vi "click.vi"(8 "error in (no error)":errorcluster, 10 "Control Label":string, 11 "VI Ref":refnum<vi>) -> (0 "error out":errorcluster, 3 "return value":string)   [LabVIEW 2020]
uses:
  ui-testing.lvlib
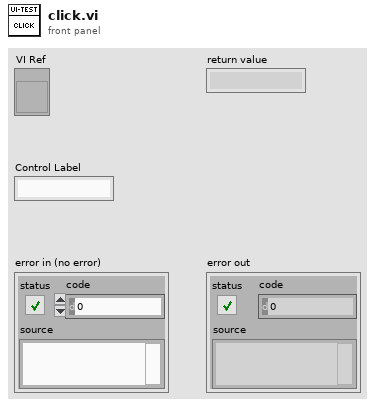
[diagram p1: front panel]
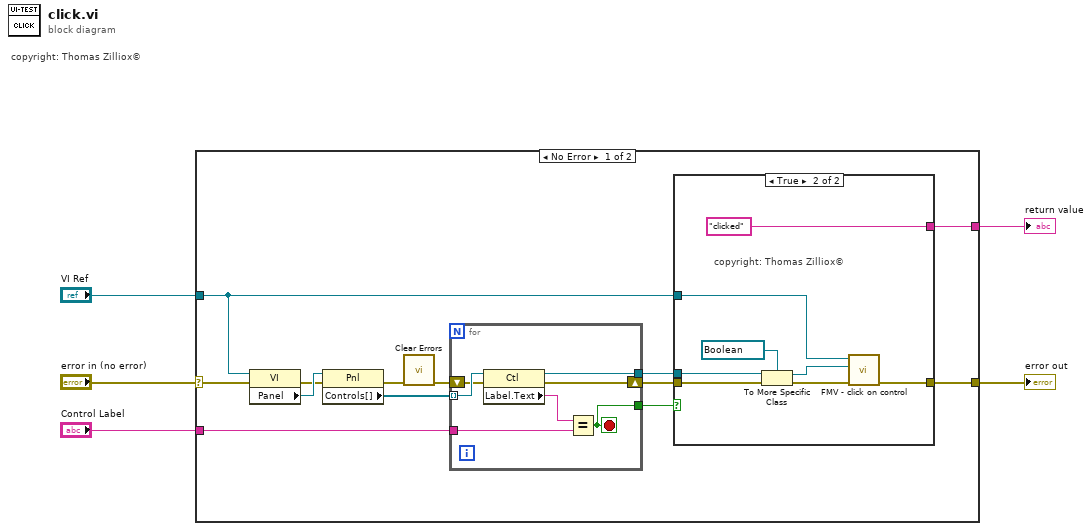
[diagram p0: block diagram]
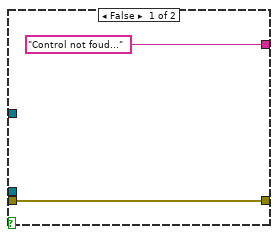
[diagram p2: hidden frame]
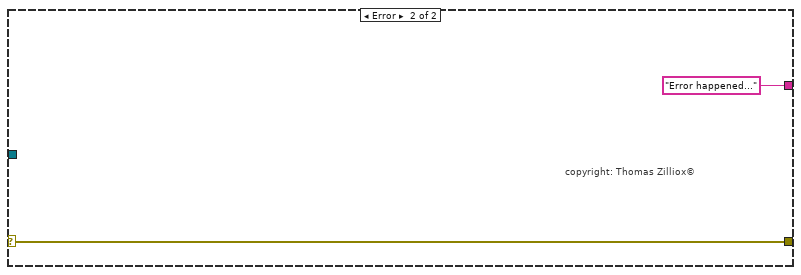
[diagram p3: hidden frame]
diagram:
  # "copyright: Thomas Zilliox©"
  n1 = case shown="No Error" "error in (no error)" {
    selector: "error in (no error)" -> [w13 w37]
    tunnel: [w11 w37] -> w4
    tunnel: "Control Label" -> [w12 _]
    tunnel: [w7 "Error happened..."] -> w2
    tunnel: "VI Ref" -> [w6 _]
    frame No Error {
      n2 = property class="VI"(reference=w6, error in=w13) -> (error out=w16:errorcluster, "Panel"=w18:refnum<vi>)  [unwired: 1 out]
      n3 = property class="Pnl"(reference=w18, error in=w16) -> (error out=w15:errorcluster, "Controls[]"=w17:refnum<vi>[])  [unwired: 1 out]
      n4 = call <vilib>:"Clear Errors.vi"("error in (no error)"=w15) -> ("error out"=w10:errorcluster)  [unwired: 5 in, 1 out]
      n5 = for {
        tunnel: w17 -> [w35] mode=indexing
        tunnel: w12 -> [w33]
        tunnel: [w32] -> w14
        shift-right: [w30] -> w9
        shift-left: w10 -> [w31]
        tunnel: [w29] -> w8
        stop <- w29 stop-if-true
        n6 = property class="Ctl"(reference=w35, error in=w31) -> (reference out=w32:refnum<vi>, error out=w30:errorcluster, "Label.Text"=w34:string)
        n7 = Equal?(x=w34, y=w33) -> (x = y?=w29:bool)
      }
      n8 = case shown="True" w8 {
        tunnel: w14 -> [_ w28]
        tunnel: w6 -> [_ w25]
        tunnel: [w19 w24] -> w11
        tunnel: w9 -> [w19 w23]
        tunnel: ["Control not foud..." "clicked" ("VI Name")] -> w7
        frame False {
        }
        frame True {
          # "copyright: Thomas Zilliox©"
          n9 = To More Specific Class(target class=refnum<vi> refnum ("Reference to Button"), reference=w28, error in=w23) -> (specific class reference=w26:refnum<vi>, error out=w22:errorcluster)
          n10 = call "FMV - click on control.vi"("error in (no error)"=w22, "Reference to Button"=w26, "VI Reference"=w25) -> ("error out"=w24:errorcluster)  [unwired: 8 in]
        }
      }
    }
    frame Error {
      # "copyright: Thomas Zilliox©"
    }
  }
  "error out" <- w4
  "return value" <- w2
